vi "Update Unmapped Channels by Filter.vi"(8 "error in (no error)":errorcluster, 11 "Loop Data in":T1) -> (0 "error out":errorcluster)   [LabVIEW 2016, in "System Mapping Tool.lvlib"]
uses:
  System Mapping Tool.lvlib
  TypeDefs/Loop Data.ctl
  TypeDefs/UI Refs.ctl
  NationalInstruments.VeriStand.SystemDefinitionAPI
  NationalInstruments.VeriStand.SystemStorageUI
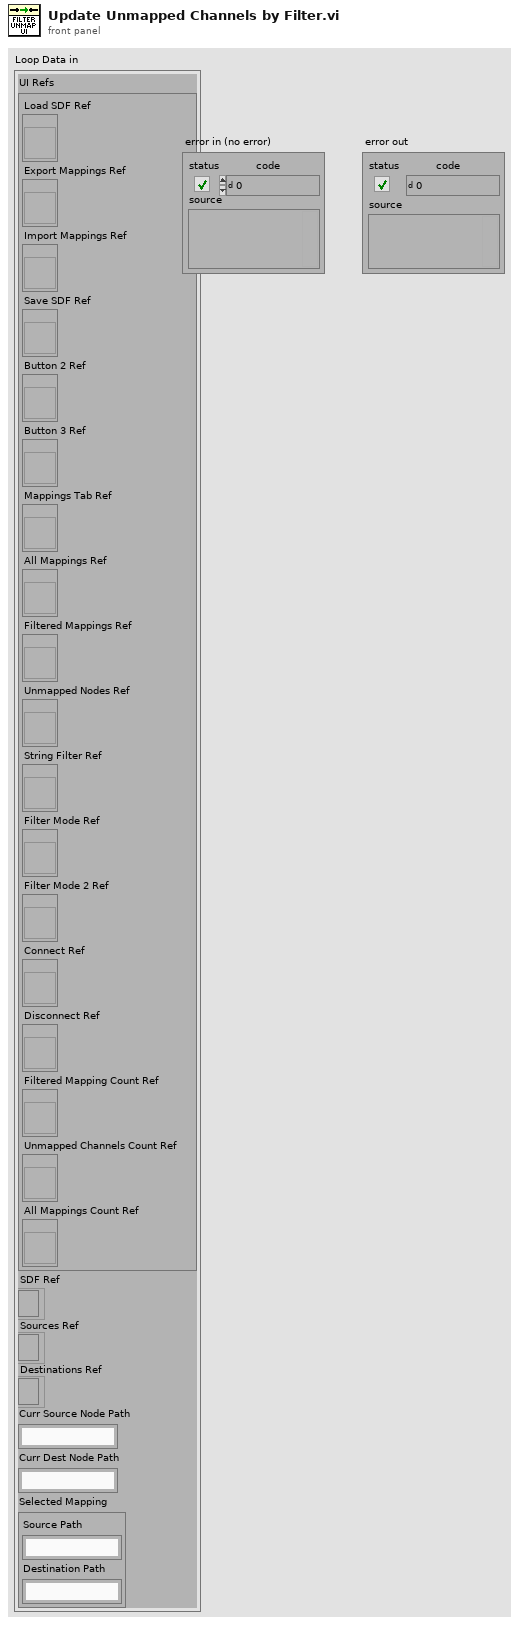
[diagram p1: front panel]
types:
  T1 = typedef "System Mapping Tool.lvlib/Loop Data.ctl" = cluster{"UI Refs":T2, "SDF Ref":refnum<k24>, "Sources Ref":refnum<k24>, "Destinations Ref":refnum<k24>, "Curr Source Node Path":string, "Curr Dest Node Path":string, "Selected Mapping":cluster{"Source Path":string, "Destination Path":string}}
  T2 = typedef "System Mapping Tool.lvlib/UI Refs.ctl" = cluster{"Load SDF Ref":refnum<vi>, "Export Mappings Ref":refnum<vi>, "Import Mappings Ref":refnum<vi>, "Save SDF Ref":refnum<vi>, "Button 2 Ref":refnum<vi>, "Button 3 Ref":refnum<vi>, "Mappings Tab Ref":refnum<vi>, "All Mappings Ref":refnum<vi>, "Filtered Mappings Ref":refnum<vi>, "Unmapped Nodes Ref":refnum<vi>, "String Filter Ref":refnum<vi>, "Filter Mode Ref":refnum<vi>, "Filter Mode 2 Ref":refnum<vi>, "Connect Ref":refnum<vi>, "Disconnect Ref":refnum<vi>, "Filtered Mapping Count Ref":refnum<vi>, "Unmapped Channels Count Ref":refnum<vi>, "All Mappings Count Ref":refnum<vi>}
  T3 = enum32{"All System Mappings", "Filtered Mappings by Node", "Unmapped Channels by Node"}
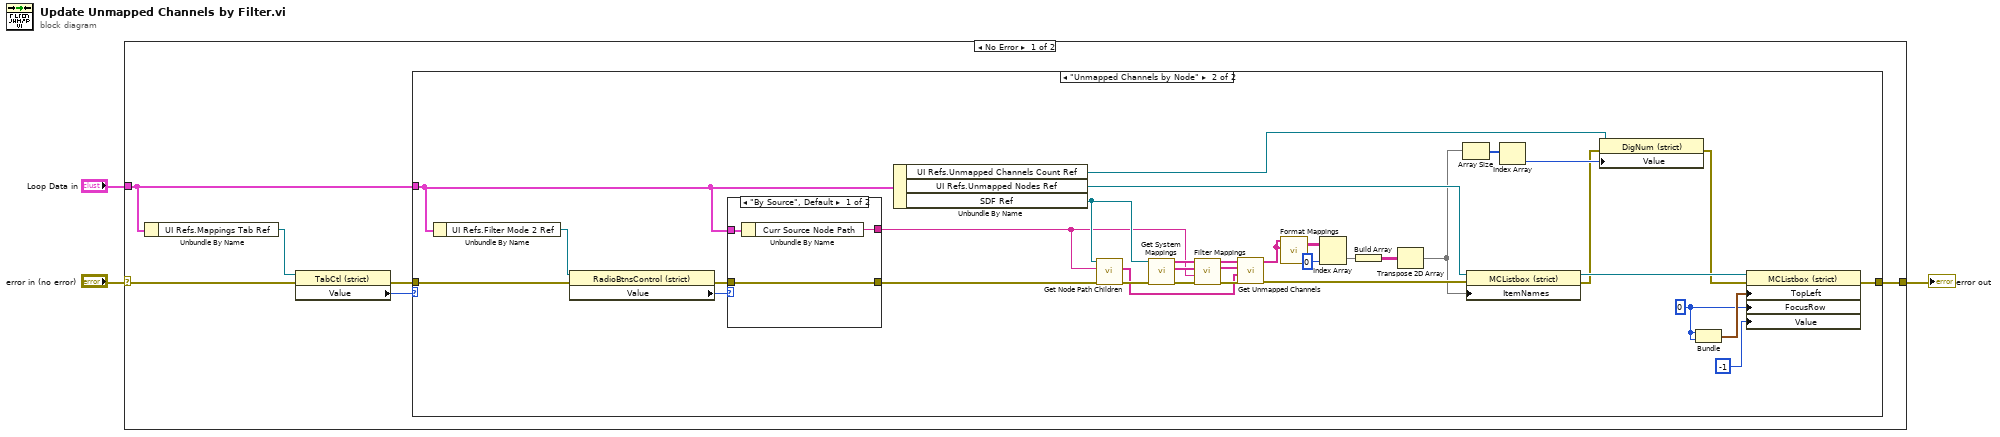
[diagram p0: block diagram]
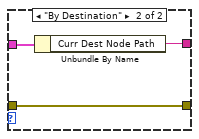
[diagram p3: hidden frame]
diagram:
  n1 = case shown="No Error" "error in (no error)" {
    selector: "error in (no error)" -> [w9 w51]
    tunnel: [w4 w51] -> w2
    tunnel: "Loop Data in" -> [w5 _]
    frame No Error {
      n2 = Unbundle By Name(w5) -> ("UI Refs.Mappings Tab Ref"=w8:refnum<vi>)
      n3 = property class="TabCtl (strict)"(reference=w8, error in=w9) -> (error out=w6:errorcluster, "Value"=w7:T3)  [unwired: 1 out]
      n4 = case shown="\"Unmapped Channels by Node\"" w7 {
        tunnel: w6 -> [w10 w44]
        tunnel: w5 -> [_ w37]
        tunnel: [w10 w35] -> w4
        frame Default {
        }
        frame "Unmapped Channels by Node" {
          w30 = 0
          n5 = Unbundle By Name(w37) -> ("UI Refs.Filter Mode 2 Ref"=w43:refnum<vi>)
          n6 = property class="RadioBtnsControl (strict)"(reference=w43, error in=w44) -> (error out=w41:errorcluster, "Value"=w42:enum32{"By Source", "By Destination"})  [unwired: 1 out]
          n7 = case shown="\"By Source\", Default" w42 {
            tunnel: w41 -> [w45 w48]
            tunnel: w37 -> [w47 w50]
            tunnel: [w46 w49] -> w19
            tunnel: [w45 w48] -> w22
            frame "By Source", Default {
              n8 = Unbundle By Name(w47) -> ("Curr Source Node Path"=w46:string)
            }
            frame "By Destination" {
              n9 = Unbundle By Name(w50) -> ("Curr Dest Node Path"=w49:string)
            }
          }
          n10 = Unbundle By Name(w37) -> ("UI Refs.Unmapped Channels Count Ref"=w14:refnum<vi>, "UI Refs.Unmapped Nodes Ref"=w36:refnum<vi>, "SDF Ref"=w20:refnum<k24>)
          n11 = call "Get Node Path Children.vi"("error in (no error)"=w22, "Node Path"=w19, "SDF Ref"=w20) -> ("error out"=w21:errorcluster, "Children"=w18:string[])  [unwired: 7 in]
          n12 = call "Get System Mappings.vi"("error in (no error)"=w21, "SDF Ref"=w20) -> ("error out"=w38:errorcluster, "Destinations"=w39:string[], "Sources"=w40:string[])  [unwired: 7 in]
          n13 = call "Filter Mappings.vi"("error in (no error)"=w38, "Path to Filter"=w19, "Destinations"=w39, "Sources"=w40) -> ("error out"=w29:errorcluster, "Filtered Destinations"=w28:string[], "Filtered Sources"=w27:string[])  [unwired: 5 in]
          n14 = call "Get Unmapped Channels.vi"("error in (no error)"=w29, "All Channels"=w18, "Destinations"=w28, "Sources"=w27) -> ("error out"=w17:errorcluster, "Unmapped Channels"=w26:string[])  [unwired: 6 in]
          n15 = call "Format Mappings.vi"("Destinations"=w26, "Sources"=w26) -> ("Mappings"=w32:string[][])  [unwired: 3 in]
          n16 = Index Array(array=w32, index (col)=0 ("disabled index (col)")) -> (element=w24:string[])  [unwired: 1 in]
          n17 = Build Array(w24) -> (w23:string[][])
          n18 = Transpose 2D Array(2D array=w23) -> (transposed array=w13:string[][])
          n19 = Array Size(array=w13) -> (size(s)=w16:i32[])
          n20 = property class="MCListbox (strict)"(reference=w36, error in=w17, "ItemNames"=w13) -> (reference out=w34:refnum<vi>, error out=w12:errorcluster)
          n21 = Index Array(array=w16) -> (element=w15:i32)  [unwired: 1 in]
          n22 = property class="DigNum (strict)"(reference=w14, error in=w12, "Value"=w15) -> (error out=w11:errorcluster)  [unwired: 1 out]
          n23 = Bundle(w30, w30) -> (w33:cluster{i32, i32})  [unwired: 1 in]
          n24 = property class="MCListbox (strict)"(reference=w34, error in=w11, "TopLeft"=w33, "FocusRow"=w30, "Value"=-1 ("index of element")) -> (error out=w35:errorcluster)  [unwired: 1 out]
        }
      }
    }
    frame Error {
    }
  }
  "error out" <- w2
